vi "Groups.vi"(8 "error in (no error)":errorcluster, 11 "Task in":refnum<class "Task.lvclass">) -> (0 "error out":errorcluster, 2 "Groups":refnum<class "GroupAbstract.lvclass">[](array[class]), 3 "Task out":refnum<class "Task.lvclass">)   [LabVIEW 2020, in "Volatus.lvlib" / "Task.lvclass"]
uses:
  Task.lvclass
  Task.lvclass/Task.ctl
  lv-vecto/Vecto/GroupAbstract/GroupAbstract.lvclass
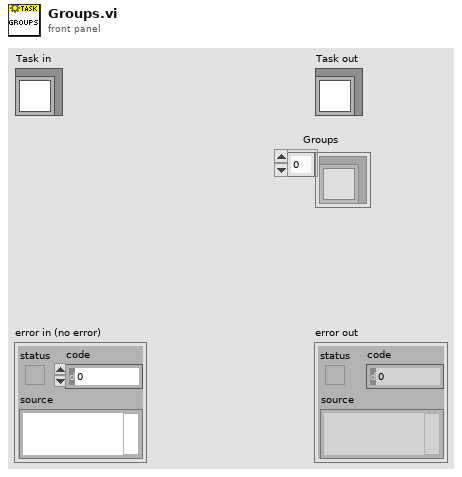
[diagram p1: front panel]
types:
  T1 = map{string, refnum<class "GroupAbstract.lvclass">}
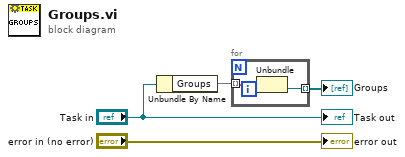
[diagram p0: block diagram]
diagram:
  n1 = Unbundle By Name("Task in") -> ("Groups"=w2:T1)
  n2 = for {
    tunnel: w2 -> [w6] mode=indexing
    tunnel: [w5] -> w1 mode=indexing
    n3 = Unbundle(w6) -> ("Group"=w5:refnum<class "GroupAbstract.lvclass">)  [unwired: 1 out]
  }
  "Groups" <- w1
  "error out" <- "error in (no error)"
  "Task out" <- "Task in"
